vi "Configure_Peak.vi"(6 "tipo_ciclo":string, 8 "error in (no error)":errorcluster, 9 "Frequency (Hz)":dbl=10.0, 10 "Amplitude (Vrms)":dbl=5.0, 11 "VISA resource name":refnum<visa-resource-name>) -> (0 "error out":errorcluster, 3 "VISA resource name out":refnum<visa-resource-name>)   [LabVIEW 2019, in "DS360.lvlib"]
uses:
  DS360.lvlib
panel:
  out "resulting string":string
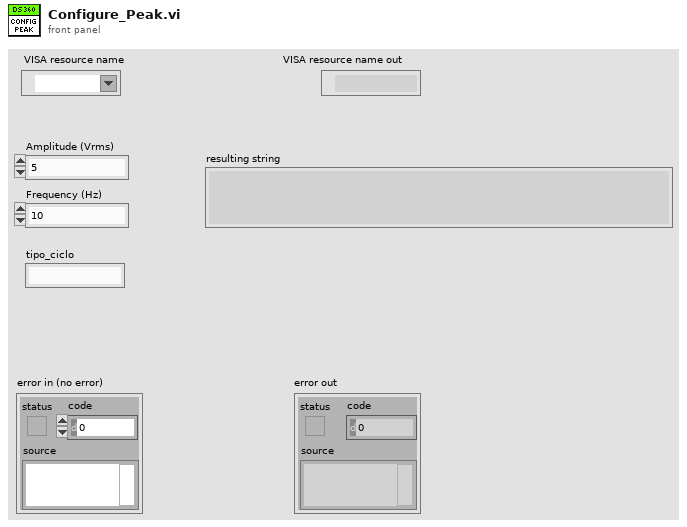
[diagram p1: front panel]
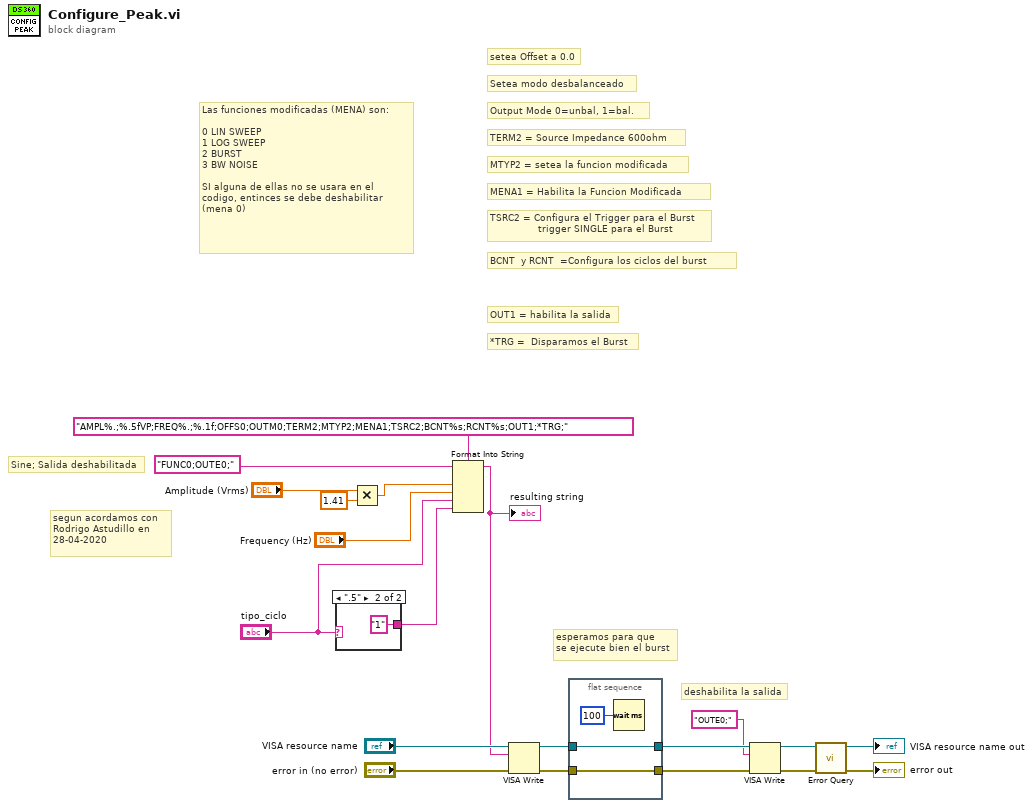
[diagram p0: block diagram]
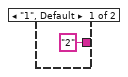
[diagram p2: hidden frame]
diagram:
  # "deshabilita la salida"
  # "esperamos para que\nse ejecute bien el burst"
  # "*TRG =  Disparamos el Burst"
  # "OUT1 = habilita la salida"
  # "BCNT  y RCNT  =Configura los ciclos del burst"
  # "TSRC2 = Configura el Trigger para el Burst\n                trigger SINGLE para el Burst"
  # "MENA1 = Habilita la Funcion Modificada"
  # "MTYP2 = setea la funcion modificada"
  # "TERM2 = Source Impedance 600ohm"
  # "Output Mode 0=unbal, 1=bal."
  # "Setea modo desbalanceado"
  # "setea Offset a 0.0"
  # "Las funciones modificadas (MENA) son:\n\n0 LIN SWEEP\n1 LOG SWEEP\n2 BURST\n3 BW NOISE\n\nSI alguna de ellas no se usara en el\ncodigo, entinces se debe deshabilitar\n(mena 0)"
  # "segun acordamos con\nRodrigo Astudillo en\n28-04-2020"
  # "Sine; Salida deshabilitada"
  n1 = case shown="\".5\"" "tipo_ciclo" {
    tunnel: ["2" ("write buffer") "1" ("write buffer")] -> w1
    frame "1", Default {
    }
    frame ".5" {
    }
  }
  n2 = Multiply(x="Amplitude (Vrms)", y=1.41) -> (x*y=w11:dbl)
  n3 = Format Into String(format string="AMPL%.;%.5fVP;FREQ%.;%.1f;OFFS0;OUTM0;TERM2;MTYP2;MENA1;TSRC2;BCNT%s;RCNT%s;OUT1;*TRG;", initial string="FUNC0;OUTE0;" ("string (\"\")"), w11, "Frequency (Hz)", "tipo_ciclo", w1) -> (resulting string=w10:string)  [unwired: 1 in, 1 out]
  "resulting string" <- w10
  n4 = VISA Write(VISA resource name="VISA resource name", write buffer=w10, error in (no error)="error in (no error)") -> (VISA resource name out=w8:refnum<visa-resource-name>, error out=w9:errorcluster)  [unwired: 1 out]
  n5 = flat-sequence {
    tunnel: w9 -> [w24]
    tunnel: [w24] -> w5
    tunnel: w8 -> [w23]
    tunnel: [w23] -> w4
    frame #0 {
      n6 = Wait (ms)(milliseconds to wait=u32 100) -> ()  [unwired: 1 out]
    }
  }
  n7 = VISA Write(VISA resource name=w4, write buffer="OUTE0;" ("string (\"\")"), error in (no error)=w5) -> (VISA resource name out=w7:refnum<visa-resource-name>, error out=w6:errorcluster)  [unwired: 1 out]
  n8 = call "Error Query.vi"("error in (no error)"=w6, "VISA resource name"=w7) -> ("error out"=→"error out":errorcluster, "VISA resource name out"=→"VISA resource name out":refnum<visa-resource-name>)  [unwired: 6 in, 2 out]
